vi "Read JPEG Files.vi"(8 "error in":errorcluster, 10 "Picture Subpanel":refnum<vi>, 11 "JPEG file path":path) -> (0 "error out":errorcluster)   [LabVIEW 2014]
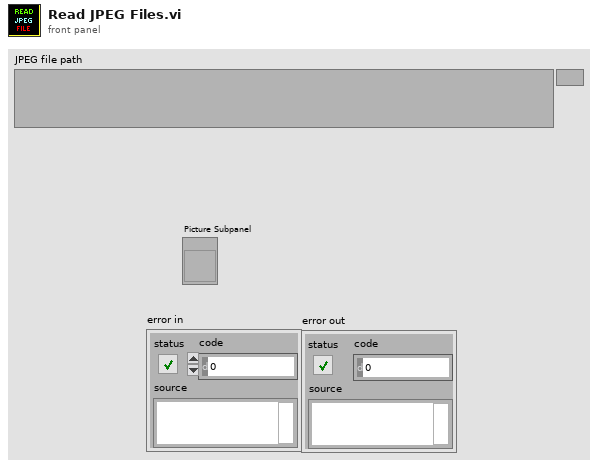
[diagram p1: front panel]
types:
  T1 = typedef "imagedata.ctl" = cluster{"image type":i32, "image depth":i32, "image":u8[], "mask":u8[], "colors":u32[], "Rectangle":cluster{"left":i16, "top":i16, "right":i16, "bottom":i16}}
  T2 = typedef "LVBoundsTypeDef.ctl" = cluster{"Width":u32, "Height":u32}
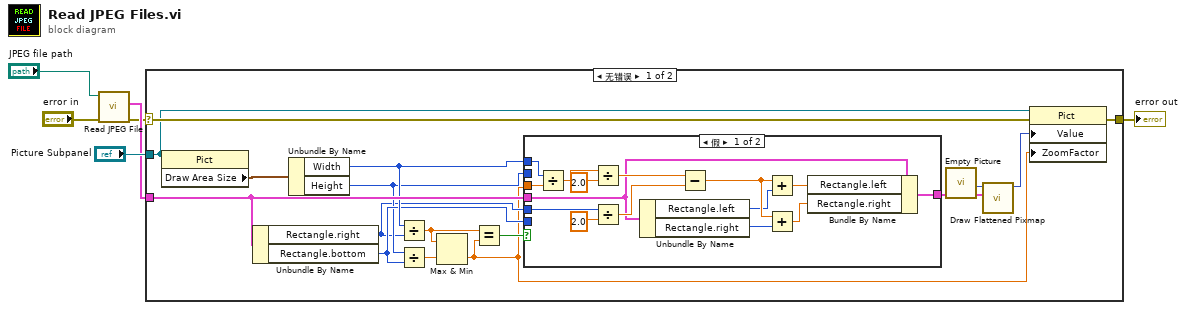
[diagram p0: block diagram]
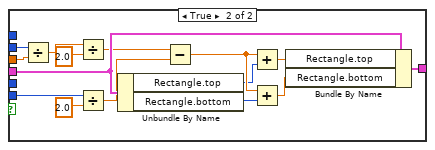
[diagram p2: hidden frame]
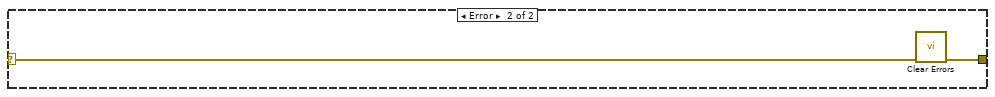
[diagram p3: hidden frame]
diagram:
  n1 = call <vilib>:"Read JPEG File.vi"("error in (no error)"="error in", "path to JPEG file"="JPEG file path") -> ("error out"=w1:errorcluster, "image data"=w2:T1)  [unwired: 7 in, 1 out]
  n2 = case shown="无错误" w1 {
    selector: w1 -> [w15 w54]
    tunnel: [w21 w53] -> w5
    tunnel: "Picture Subpanel" -> [w13 _]
    tunnel: w2 -> [w18 _]
    frame No Error {
      n3 = property class="Pict"(reference=w13) -> ("Draw Area Size"=w14:T2)  [unwired: 1 in, 2 out]
      n4 = Unbundle By Name(w18) -> ("Rectangle.right"=w8:i16, "Rectangle.bottom"=w11:i16)
      n5 = Unbundle By Name(w14) -> ("Width"=w12:u32, "Height"=w10:u32)
      n6 = Divide(x=w12, y=w8) -> (x/y=w20:dbl)
      n7 = Divide(x=w10, y=w11) -> (x/y=w16:dbl)
      n8 = Max & Min(x=w20, y=w16) -> (min(x,y)=w7:dbl)  [unwired: 1 out]
      n9 = Equal?(x=w20, y=w7) -> (x = y?=w19:bool)
      n10 = case shown="假" w19 {
        tunnel: w11 -> [_ w49]
        tunnel: w18 -> [w27 w51]
        tunnel: [w26 w50] -> w17
        tunnel: w7 -> [w23 w48]
        tunnel: w12 -> [w25 _]
        tunnel: w10 -> [_ w52]
        tunnel: w8 -> [w24 _]
        frame False {
          n11 = Divide(x=w25, y=w23) -> (x/y=w36:dbl)
          n12 = Divide(x=w36, y=2.0) -> (x/y=w34:dbl)
          n13 = Divide(x=w24, y=2.0) -> (x/y=w33:dbl)
          n14 = Unbundle By Name(w27) -> ("Rectangle.left"=w28:i16, "Rectangle.right"=w30:i16)
          n15 = Subtract(x=w34, y=w33) -> (x-y=w32:dbl)
          n16 = Add(x=w32, y=w28) -> (x+y=w29:dbl)
          n17 = Add(x=w32, y=w30) -> (x+y=w31:dbl)
          n18 = Bundle By Name(cluster=w27, "Rectangle.left"=w29, "Rectangle.right"=w31) -> (w26:T1)
        }
        frame True {
          n19 = Divide(x=w52, y=w48) -> (x/y=w46:dbl)
          n20 = Divide(x=w46, y=2.0) -> (x/y=w44:dbl)
          n21 = Divide(x=w49, y=2.0) -> (x/y=w43:dbl)
          n22 = Unbundle By Name(w51) -> ("Rectangle.top"=w38:i16, "Rectangle.bottom"=w40:i16)
          n23 = Subtract(x=w44, y=w43) -> (x-y=w42:dbl)
          n24 = Add(x=w42, y=w38) -> (x+y=w39:dbl)
          n25 = Add(x=w42, y=w40) -> (x+y=w41:dbl)
          n26 = Bundle By Name(cluster=w51, "Rectangle.top"=w39, "Rectangle.bottom"=w41) -> (w50:T1)
        }
      }
      n27 = call "Empty Picture"() -> ("empty picture"=w22:picture)
      n28 = call <vilib>:"Draw Flattened Pixmap.vi"("image data"=w17, "picture"=w22) -> ("new picture"=w9:picture)  [unwired: 7 in]
      n29 = property class="Pict"(reference=w13, error in=w15, "Value"=w9, "ZoomFactor"=w7) -> (error out=w21:errorcluster)  [unwired: 1 out]
    }
    frame Error {
      n30 = call <vilib>:"Clear Errors.vi"("error in (no error)"=w54) -> ("error out"=w53:errorcluster)  [unwired: 5 in, 1 out]
    }
  }
  "error out" <- w5
